vi "Get_Calib_zero_Offset.vi"(1 "Measurement Time":dbl format="%#.0f", 2 "Calib Filename":path) -> (0 "Voltage Offset":dbl)   [LabVIEW 2017]
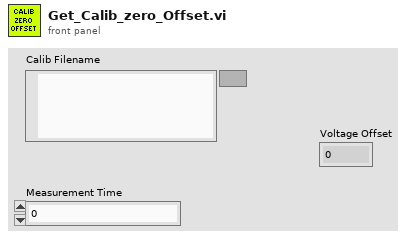
[diagram p1: front panel]
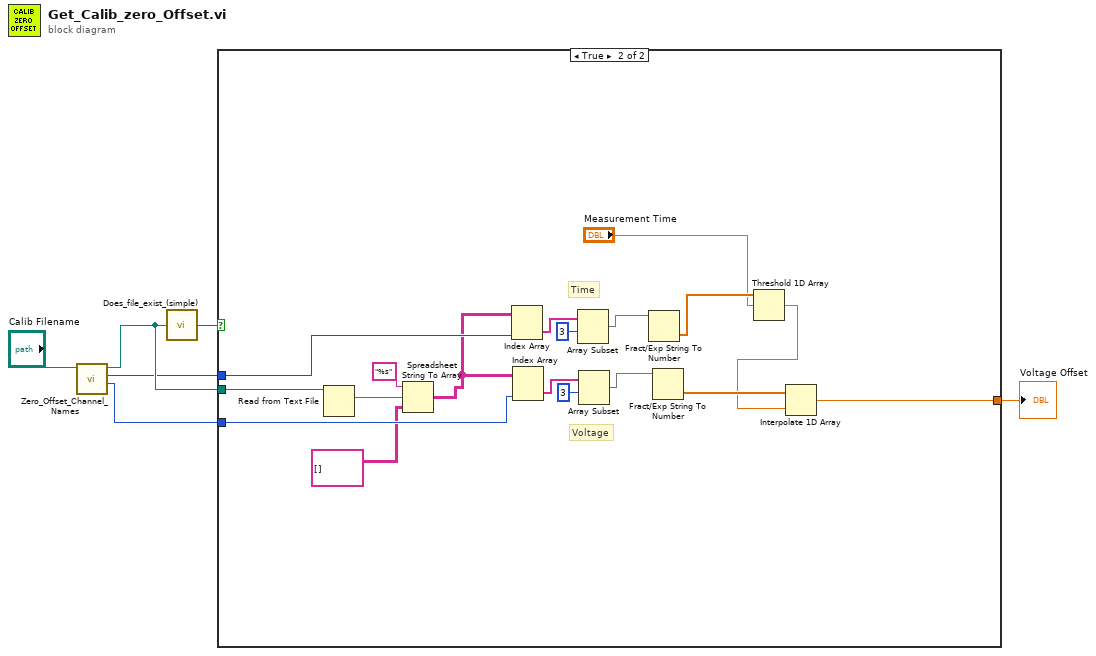
[diagram p0: block diagram]
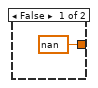
[diagram p2: hidden frame]
diagram:
  n1 = call "Zero_Offset_Channel_Names.vi"("Calib Filename"="Calib Filename") -> ("Voltage Index"=w2:i32, "Time Index"=w3:i32, "Zero Filename"=w4:path)  [unwired: 3 in, 1 out]
  n2 = call "Does_file_exist_(simple).vi"("Pathname"=w4) -> ("exists?"=w5:bool)
  n3 = case shown="True" w5 {
    tunnel: w4 -> [_ w25]
    tunnel: w3 -> [_ w23]
    tunnel: w2 -> [_ w17]
    tunnel: [nan w8] -> w1
    frame False {
    }
    frame True {
      # "Voltage"
      # "Time"
      n4 = Read from Text File(file (use dialog)=w25) -> (text=w24:string)  [unwired: 3 in, 3 out]
      n5 = Spreadsheet String To Array(format string="%s", spreadsheet string=w24, array type (2D Dbl)=string[][] []) -> (array=w18:string[][])  [unwired: 1 in]
      n6 = Index Array(array=w18, index (col)=w23) -> (element=w22:string[])  [unwired: 1 in]
      n7 = Index Array(array=w18, index (col)=w17) -> (element=w19:string[])  [unwired: 1 in]
      n8 = Array Subset(array=w22, index=3) -> (w14:string[])  [unwired: 1 in]
      n9 = Array Subset(array=w19, index=3) -> (w11:string[])  [unwired: 1 in]
      n10 = Fract/Exp String To Number(string=w14) -> (number=w13:dbl[])  [unwired: 3 in, 1 out]
      n11 = Fract/Exp String To Number(string=w11) -> (number=w10:dbl[])  [unwired: 3 in, 1 out]
      n12 = Threshold 1D Array(2:"Measurement Time", 3:w13) -> (0:w9:dbl)  [unwired: 1 in]
      n13 = Interpolate 1D Array(1:w9, 2:w10) -> (0:w8:dbl)
    }
  }
  "Voltage Offset" <- w1
